vi "Repace Empty String.vi"(7 "EmptyRepaceString":string, 11 "String In":string) -> (3 "String Out":string)   [LabVIEW 2021]
doc: "if input string is empyt , output Idle or customer input string"
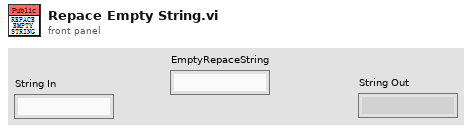
[diagram p1: front panel]
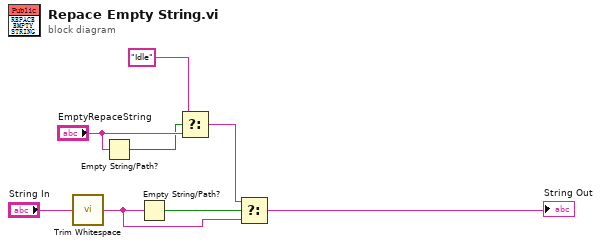
[diagram p0: block diagram]
diagram:
  n1 = call <vilib>:"Trim Whitespace.vi"("string"="String In") -> ("trimmed string"=w6:string)  [unwired: 1 in]
  n2 = Empty String/Path?(string/path="EmptyRepaceString") -> (empty?=w1:bool)
  n3 = Empty String/Path?(string/path=w6) -> (empty?=w7:bool)
  n4 = Select(t="Idle", s=w1, f="EmptyRepaceString") -> (s? t:f=w3:string)
  n5 = Select(t=w3, s=w7, f=w6) -> (s? t:f=→"String Out":string)
